vi "GetTemperature.vi"(4 "Device":u8=1, 5 "Serial port":refnum<visa-resource-name>) -> (0 "Temperature":sgl, 1 "Device out":u8=1, 2 "Serial port out":refnum<visa-resource-name>)   [LabVIEW 2021]
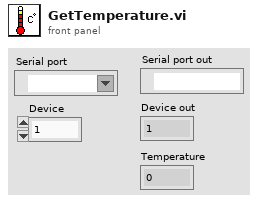
[diagram p1: front panel]
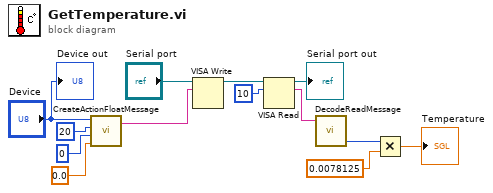
[diagram p0: block diagram]
diagram:
  n1 = call "CreateActionFloatMessage.vi"("Value"=sgl 0.0, "Key"=u32 0, "Action"=u8 20, "Device"="Device") -> ("Message"=w7:string)  [unwired: 1 in]
  n2 = VISA Write(VISA resource name="Serial port", write buffer=w7) -> (VISA resource name out=w13:refnum<visa-resource-name>)  [unwired: 1 in, 2 out]
  n3 = VISA Read(VISA resource name=w13, byte count=u32 10) -> (VISA resource name out=→"Serial port out":refnum<visa-resource-name>, read buffer=w3:string)  [unwired: 1 in, 2 out]
  n4 = call "DecodeReadMessage.vi"("Message"=w3) -> ("Value"=w2:i32)  [unwired: 2 in, 2 out]
  n5 = Multiply(x=w2, y=sgl 0.0078125) -> (x*y=→"Temperature":sgl)
  "Device out" <- "Device"
